vi "RF Reader (Host).vi"() -> ()   [LabVIEW 2018]
panel:
  in  "stop":bool
  in  "Next Frame":bool
  out "progress":dbl(slide) scale=0.0..100.0
  in  "indicator tab":enum32{"Power Spectrum", "I & Q Data"}(tab)
  out "power spectrum":cluster{"f0":dbl, "df":dbl, "magnitude":dbl[]}(graph) caption="Power Spectrum"
  out "iq data":waveform(dbl)[](graph) caption="I & Q Data"
  in  "Frame length, samples":i32
  in  "Rec file":path
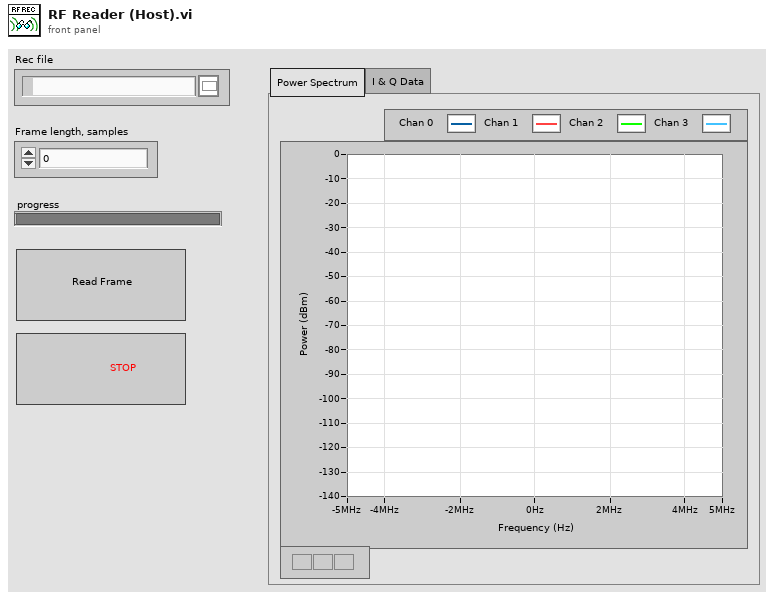
[diagram p1: front panel]
types:
  T1 = enum16{"open", "replace", "create", "open or create", "replace or create", "replace or create with confirmation"}
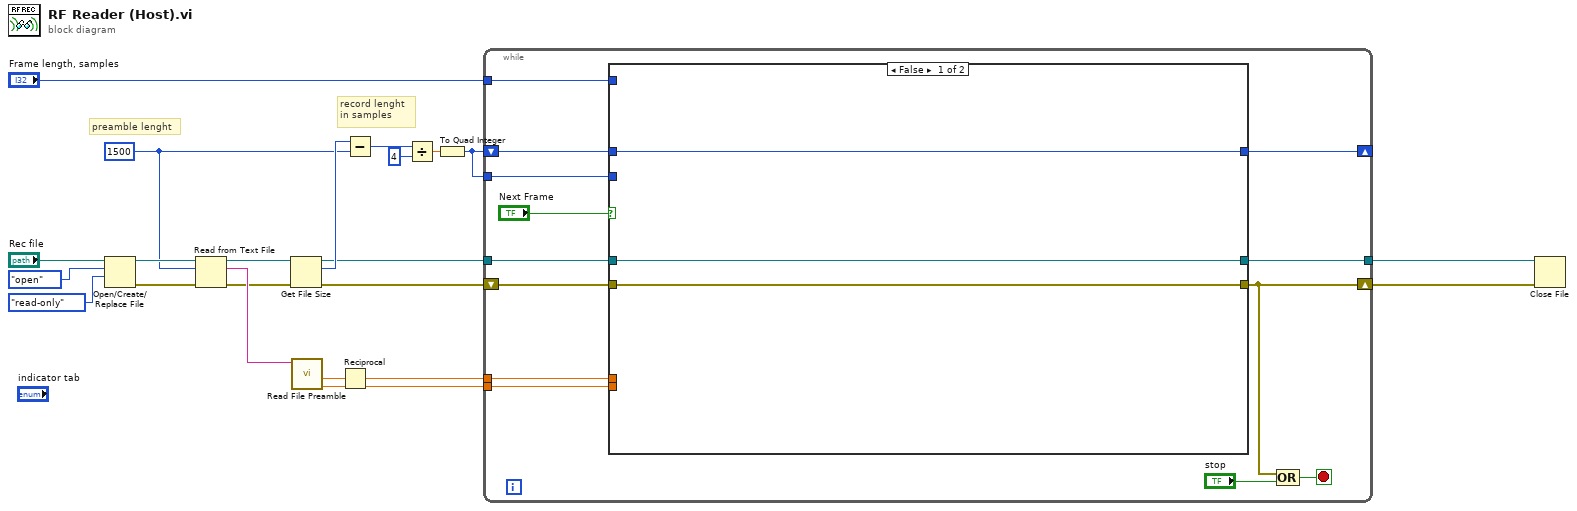
[diagram p0: block diagram]
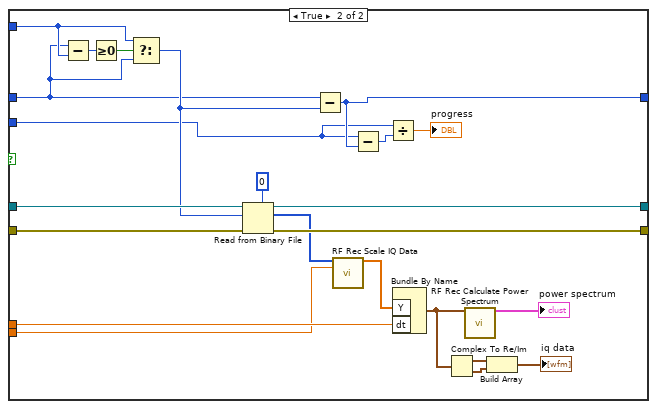
[diagram p2: hidden frame]
diagram:
  w10 = 1500 ("count")
  # "record lenght \nin samples"
  # "preamble lenght"
  n1 = Open/Create/Replace File(file path (use dialog)="Rec file", operation (0:open)=T1."open", access (0:read/write)=enum16{"read/write", "read-only", "write-only"}."read-only") -> (refnum out=w19:refnum<file>, error out=w18:errorcluster)  [unwired: 3 in, 1 out]
  n2 = Read from Text File(file (use dialog)=w19, count=w10, error in=w18) -> (refnum out=w13:refnum<file>, text=w17:string, error out=w12:errorcluster)  [unwired: 1 in, 1 out]
  n3 = Get File Size(file=w13, error in=w12) -> (refnum out=w9:refnum<file>, size (in bytes)=w11:i64, 0:w8:errorcluster)
  n4 = call "Read File Preamble.vi"("file preamble"=w17) -> ("vertical range"=w1:dbl, "sample rate"=w3:dbl)  [unwired: 7 in, 2 out]
  n5 = Reciprocal(x=w3) -> (1/x=w2:dbl)
  n6 = Subtract(x=w11, y=w10) -> (x-y=w7:i64)
  n7 = Divide(x=w7, y=i64 4) -> (x/y=w5:dbl)
  n8 = To Quad Integer(1:w5) -> (0:w4:i64)
  n9 = while {
    tunnel: w9 -> [w35]
    tunnel: "Frame length, samples" -> [w32]
    tunnel: [w33] -> w15
    shift-right: [w23] -> w14
    shift-left: w8 -> [w34]
    shift-right: [w30] -> _
    shift-left: w4 -> [w31]
    tunnel: w4 -> [w29]
    tunnel: w2 -> [w28]
    tunnel: w1 -> [w27]
    stop <- w24 stop-if-true
    n10 = case shown="False" "Next Frame" {
      tunnel: w35 -> [w38 w61]
      tunnel: w34 -> [w36 w59]
      tunnel: [w38 w58] -> w33
      tunnel: [w36 w57] -> w23
      tunnel: w32 -> [_ w53]
      tunnel: w31 -> [w37 w51]
      tunnel: [w37 w50] -> w30
      tunnel: w29 -> [_ w48]
      tunnel: w28 -> [_ w45]
      tunnel: w27 -> [_ w44]
      frame False {
      }
      frame True {
        n11 = Subtract(x=w51, y=w53) -> (x-y=w55:i64)
        n12 = Greater Or Equal To 0?(x=w55) -> (x >= 0?=w54:bool)
        n13 = Select(t=w53, s=w54, f=w51) -> (s? t:f=w52:i64)
        n14 = Read from Binary File(5:u32 0, 8:w59, 10:w52, 11:w61) -> (0:w57:errorcluster, 2:w56:u32[], 3:w58:refnum<file>)  [unwired: 2 in, 1 out]
        n15 = Subtract(x=w51, y=w52) -> (x-y=w50:i64)
        n16 = call "RF Rec Scale IQ Data.vi"("raw waveform data"=w56, "scaling (V/code)"=w44) -> ("scaled data"=w46:cdb[])  [unwired: 13 in]
        n17 = Subtract(x=w48, y=w50) -> (x-y=w49:i64)
        n18 = Divide(x=w48, y=w49) -> (x/y=→"progress":dbl)
        n19 = Bundle By Name("Y"=w46, "dt"=w45) -> (w40:waveform(cdb))  [unwired: 1 in]
        n20 = Complex To Re/Im(x + iy=w40) -> (x=w42:waveform(dbl), y=w41:waveform(dbl))
        n21 = call "RF Rec Calculate Power Spectrum.vi"("waveform"=w40) -> ("power spectrum (dBm)"=→"power spectrum":cluster{"f0":dbl, "df":dbl, "magnitude":dbl[]})  [unwired: 14 in]
        n22 = Build Array(w42, w41) -> (→"iq data":waveform(dbl)[])
      }
    }
    n23 = Compound Arithmetic op=OR(w23, "stop") -> (w24:bool)
  }
  n24 = Close File(refnum=w15, error in=w14) -> ()  [unwired: 2 out]
